vi "Get Target Method Icon.vi"(8 "error in (no error)":errorcluster, 10 "Target Method path":path, 11 "Application in":refnum<vi>) -> (0 "error out":errorcluster, 1 "Icon out":refnum<class "Icon.lvclass">)   [LabVIEW 2020, in "Message Maker.lvlib"]
uses:
  Message Maker.lvlib
  <vilib>/LabVIEW Icon API/LabVIEW Icon API.lvlib
  <vilib>/picture/picture.llb/imagedata.ctl
  <vilib>/Utility/miscctls.llb/LVPoint32TypeDef.ctl
  <vilib>/LabVIEW Icon API/API_User Layer Data.ctl
  Localized Strings.vi
  <vilib>/LabVIEW Icon API/lv_icon/Classes/Icon/Icon.lvclass
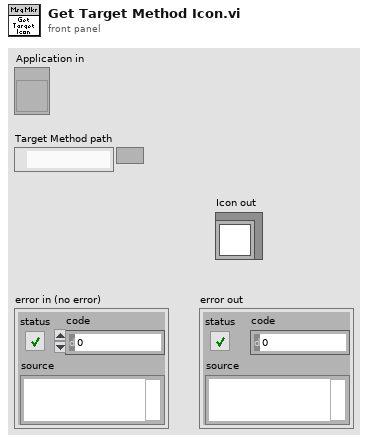
[diagram p1: front panel]
types:
  T1 = typedef "LabVIEW Icon API.lvlib/API_User Layer Data.ctl" = cluster{"Layer name":string, "Origin":T2, "Icon image data":T3}
  T2 = typedef "LVPoint32TypeDef.ctl" = cluster{"Horizontal":i32, "Vertical":i32}
  T3 = typedef "imagedata.ctl" = cluster{"image type":i32, "image depth":i32, "image":u8[], "mask":u8[], "colors":u32[], "Rectangle":cluster{"left":i16, "top":i16, "right":i16, "bottom":i16}}
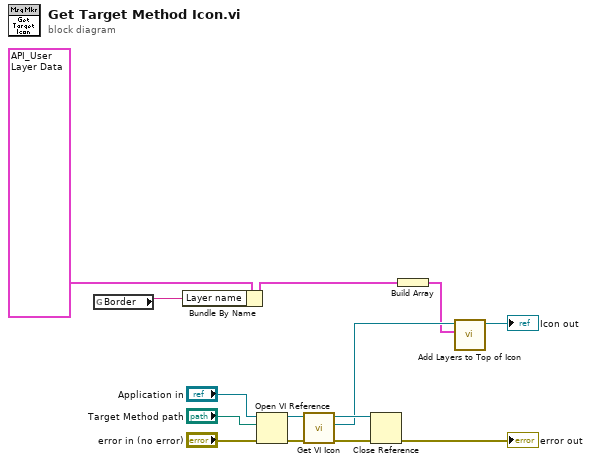
[diagram p0: block diagram]
diagram:
  n1 = global read "Localized Strings.vi" "Border"() -> (w1:string)
  n2 = Bundle By Name(cluster=T1 {"Layer name"="Border", "Origin"={"Horizontal"=0, "Vertical"=0}, "Icon image data"={"image type"=0, "image depth"=24, "image"=array[3072 elements], "mask"=[], "colors"=[], "Rectangle"={"left"=0, "top"=0, "right"=32, "bottom"=32}}} ("User Layer data"), "Layer name"=w1) -> (w2:T1)
  n3 = Open VI Reference(application reference (local)="Application in", vi path="Target Method path", error in (no error)="error in (no error)") -> (vi reference=w11:refnum<vi>, error out=w12:errorcluster)  [unwired: 3 in]
  n4 = call <vilib>:"Get VI Icon.vi"("error in (no error)"=w12, "VI Refnum in"=w11) -> ("error out"=w8:errorcluster, "Icon"=w7:refnum<class "Icon.lvclass">, "VI Refnum out"=w13:refnum<vi>)  [unwired: 7 in]
  n5 = Close Reference(reference=w13, error in (no error)=w8) -> (error out=→"error out":errorcluster)
  n6 = Build Array(w2) -> (w3:T1[])
  n7 = call "Add Layers to Top of Icon.vi"("User layers"=w3, "Icon.lvclass in"=w7) -> ("Icon.lvclass out"=→"Icon out":refnum<class "Icon.lvclass">)  [unwired: 9 in]
